vi "Overlord.vi"(0 "Pathfinding Settings":T1={"Movement Settings"={"Arrival Tolerance (m)"=0.01, "Closeness Threshold (m)"=0.5, "Pit Obstacle Radius (m)"=0.5, "Pit Locations"=[]}, "Dead Zone"=0.75, "Max Moves"=2.0, "Move Segment Length (m)"=0.2, "Path Cost Weights"={"Length Weight"=1.0, "Angle Weight"=0.0, "Angle Error Weight"=1000.0, "Angle Error Threshold"=0.314, "Per Move Penalty"=0.05, "Closeness Weight"=100.0, "Too Short Penalty"=100.0, "Too Short Threshold"=1.5}, "Desperation - Reduction Per Attempt (Ratio)"=0.9, "Desperation - Max Attempts"=1, "Log All Move Points"=TRUE, "Intermediate Position Grids"=[{"x1"=0.0, "x2"=1.75, "resolution"=0.15}, {"x1"=1.75, "x2"=7.38, "resolution"=0.4}]}) -> ()   [LabVIEW 2015, in "Overlord2017.lvlib"]
doc: "Note: pathfinding settings not required. This VI can run headless. Set default values before deploying to myRIO."
uses:
  Overlord2017.lvlib
  PathfindingSettings.ctl
  MovementSettings.ctl
  PathCostWeights.ctl
  IntermediatePositionGrids.ctl
  Navigation2017.lvlib
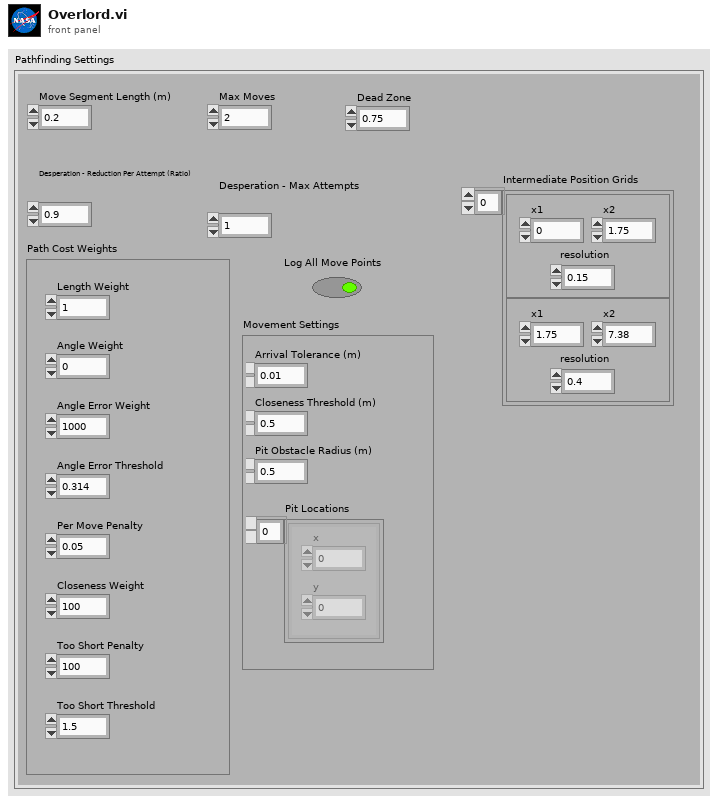
[diagram p1: front panel]
types:
  T1 = typedef "Navigation2017.lvlib/PathfindingSettings.ctl" = cluster{"Movement Settings":T2, "Dead Zone":dbl, "Max Moves":dbl, "Move Segment Length (m)":dbl, "Path Cost Weights":T3, "Desperation - Reduction Per Attempt (Ratio)":dbl, "Desperation - Max Attempts":i16, "Log All Move Points":bool, "Intermediate Position Grids":T4}
  T2 = typedef "Navigation2017.lvlib/MovementSettings.ctl" = cluster{"Arrival Tolerance (m)":dbl, "Closeness Threshold (m)":dbl, "Pit Obstacle Radius (m)":dbl, "Pit Locations":cluster{"x":dbl, "y":dbl}[]}
  T3 = typedef "Navigation2017.lvlib/PathCostWeights.ctl" = cluster{"Length Weight":dbl, "Angle Weight":dbl, "Angle Error Weight":dbl, "Angle Error Threshold":dbl, "Per Move Penalty":dbl, "Closeness Weight":dbl, "Too Short Penalty":dbl, "Too Short Threshold":dbl}
  T4 = typedef "Navigation2017.lvlib/IntermediatePositionGrids.ctl" = cluster{"x1":dbl, "x2":dbl, "resolution":dbl}[]
  T5 = enum16{"Spin and Move To Mining Area", "Move To Collector Trough", "Move To Mining Area"}
  T6 = typedef "LocalizationStatus.ctl" = cluster{"x":dbl, "y":dbl, "angle":dbl, "valid":bool, "lastUpdatedTime":dbl}
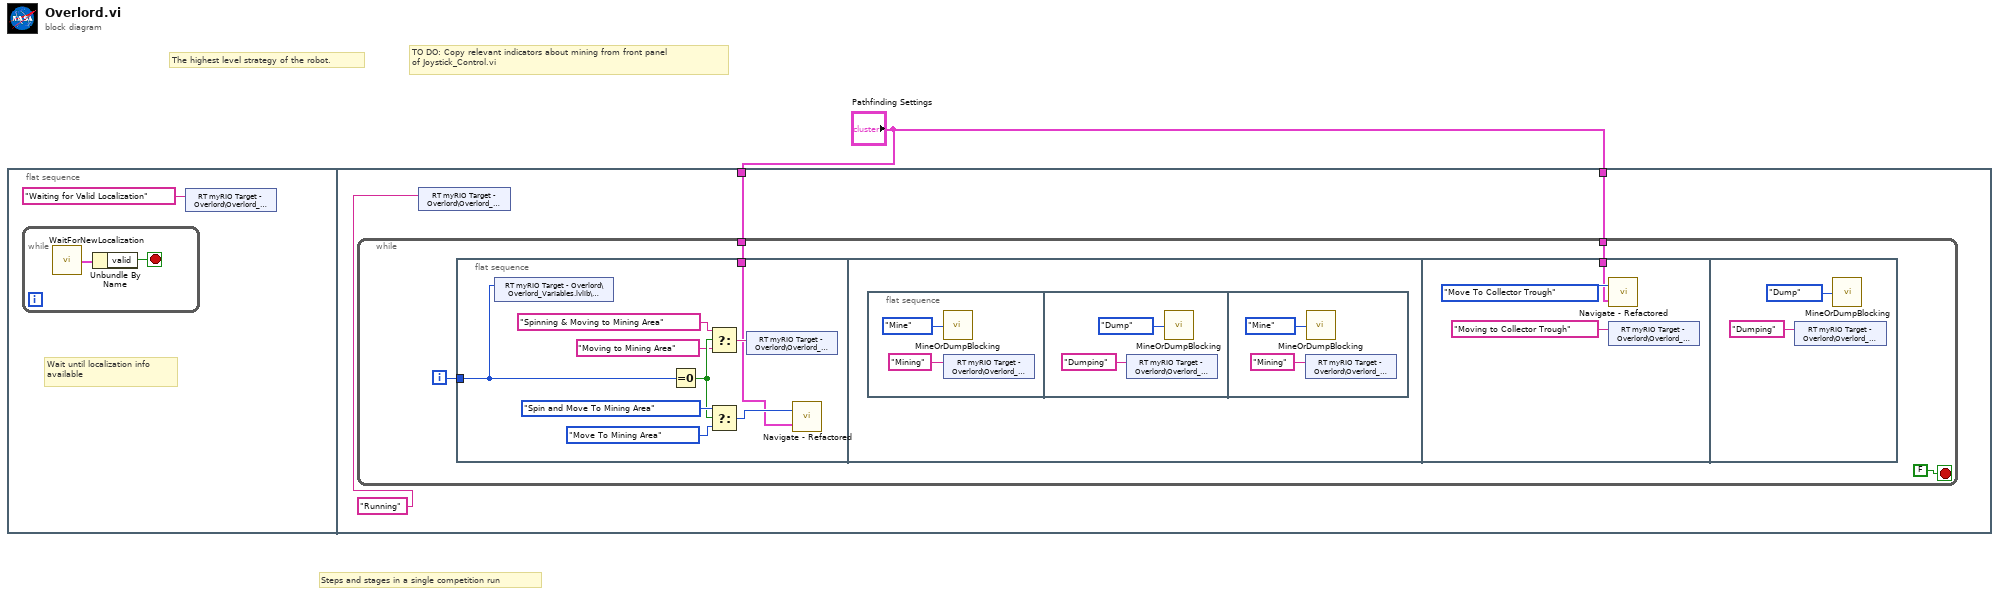
[diagram p0: block diagram]
diagram:
  # "The highest level strategy of the robot."
  # "Steps and stages in a single competition run"
  # "TO DO: Copy relevant indicators about mining from front panel\nof Joystick_Control.vi"
  n1 = flat-sequence {
    tunnel: "Pathfinding Settings" -> [w6]
    tunnel: "Pathfinding Settings" -> [w5]
    frame #0 {
      # "Wait until localization info\navailable"
      n2 = while {
        stop <- w4 stop-if-true
        n3 = call "WaitForNewLocalization.vi"() -> ("Localization Status"=w3:T6)
        n4 = Unbundle By Name(w3) -> ("valid"=w4:bool)
      }
      n5 = shared-variable "RT myRIO Target - Overlord\\Overlord_Variables.lvlib\\CurrStage"("Waiting for Valid Localization" ("CurrStage")) -> ()  [unwired: 1 in, 1 out]
    }
    frame #1 {
      n6 = while {
        tunnel: w6 -> [w9]
        tunnel: w5 -> [w8]
        i -> [w11]
        stop <- FALSE stop-if-true
        n7 = flat-sequence {
          tunnel: w11 -> [w13]
          tunnel: w9 -> [w12]
          tunnel: w8 -> [w27]
          frame #0 {
            n8 = shared-variable "RT myRIO Target - Overlord\\Overlord_Variables.lvlib\\CurrMiningRun"(w13) -> ()  [unwired: 1 in, 1 out]
            n9 = Equal To 0?(x=w13) -> (x = 0?=w15:bool)
            n10 = Select(t="Spinning & Moving to Mining Area" ("CurrStage"), s=w15, f="Moving to Mining Area") -> (s? t:f=w17:string)
            n11 = Select(t=T5."Spin and Move To Mining Area" ("Move Type"), s=w15, f=T5."Move To Mining Area") -> (s? t:f=w18:T5)
            n12 = shared-variable "RT myRIO Target - Overlord\\Overlord_Variables.lvlib\\CurrStage"(w17) -> ()  [unwired: 1 in, 1 out]
            n13 = call "Navigate - Refactored.vi"("Pathfinding Settings"=w12, "Move Type"=w18) -> ()  [unwired: 1 in]
          }
          frame #1 {
            n14 = flat-sequence {
              frame #0 {
                n15 = call "MineOrDumpBlocking.vi"("Action"=enum16{"Dump", "Mine"}."Mine") -> ()
                n16 = shared-variable "RT myRIO Target - Overlord\\Overlord_Variables.lvlib\\CurrStage"("Mining" ("CurrStage")) -> ()  [unwired: 1 in, 1 out]
              }
              frame #1 {
                n17 = shared-variable "RT myRIO Target - Overlord\\Overlord_Variables.lvlib\\CurrStage"("Dumping" ("CurrStage")) -> ()  [unwired: 1 in, 1 out]
                n18 = call "MineOrDumpBlocking.vi"("Action"=enum16{"Dump", "Mine"}."Dump") -> ()
              }
              frame #2 {
                n19 = shared-variable "RT myRIO Target - Overlord\\Overlord_Variables.lvlib\\CurrStage"("Mining" ("CurrStage")) -> ()  [unwired: 1 in, 1 out]
                n20 = call "MineOrDumpBlocking.vi"("Action"=enum16{"Dump", "Mine"}."Mine") -> ()
              }
            }
          }
          frame #2 {
            n21 = call "Navigate - Refactored.vi"("Pathfinding Settings"=w27, "Move Type"=T5."Move To Collector Trough") -> ()  [unwired: 1 in]
            n22 = shared-variable "RT myRIO Target - Overlord\\Overlord_Variables.lvlib\\CurrStage"("Moving to Collector Trough" ("CurrStage")) -> ()  [unwired: 1 in, 1 out]
          }
          frame #3 {
            n23 = shared-variable "RT myRIO Target - Overlord\\Overlord_Variables.lvlib\\CurrStage"("Dumping" ("CurrStage")) -> ()  [unwired: 1 in, 1 out]
            n24 = call "MineOrDumpBlocking.vi"("Action"=enum16{"Dump", "Mine"}."Dump") -> ()
          }
        }
      }
      n25 = shared-variable "RT myRIO Target - Overlord\\Overlord_Variables.lvlib\\CurrStage"("Running" ("CurrStage")) -> ()  [unwired: 1 in, 1 out]
    }
  }
